vi "Read Mulit Voltage.vi"() -> ()   [LabVIEW 2019]
uses:
  BRC-DAQ.lvlib
panel:
  out "get parameters":T1={"Sample Rate"=51200.0, "Coupling Model"=1, "IEPE Current(mA)"=4.0} {"IEPE Current(mA)" format="%#_13g"; "Coupling Model" items=["DC", "AC"]; "Sample Rate" format="%#_13g"}
  out "Numeric":i32
  in  "Stop":bool
  out "Waveform Graph":waveform(dbl)[](graph)
  in  "set parameters":T1={"Sample Rate"=51200.0, "Coupling Model"=1, "IEPE Current(mA)"=4.0} {"IEPE Current(mA)" format="%#_13g"; "Coupling Model" items=["DC", "AC"]; "Sample Rate" format="%#_13g"}
  in  "Physical ID":i32
  out "Module Information":cluster{"ID":string, "Name":string, "CH":i32}[](array[cluster])
  in  "rawValue":bool
  # "Channel Setting"
  # "Acquired Data"
  # "Acquired Parameters"
  # "Module Parameters"
  # "Module Information"
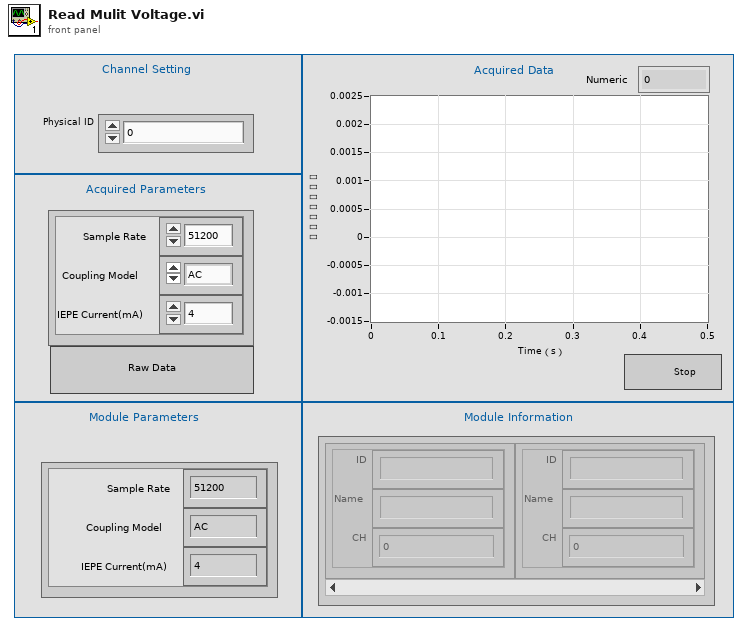
[diagram p1: front panel]
types:
  T1 = cluster{"Sample Rate":dbl, "Coupling Model":i32, "IEPE Current(mA)":dbl}
  T2 = typedef "BRC-DAQ.lvlib/brc_daq_pModuleInfo.ctl" = cluster{"deviceId":string, "productName":string, "channelCount":i32}
  T3 = cluster{"sample_rate":dbl, "coupling_mode":i32, "current":dbl}
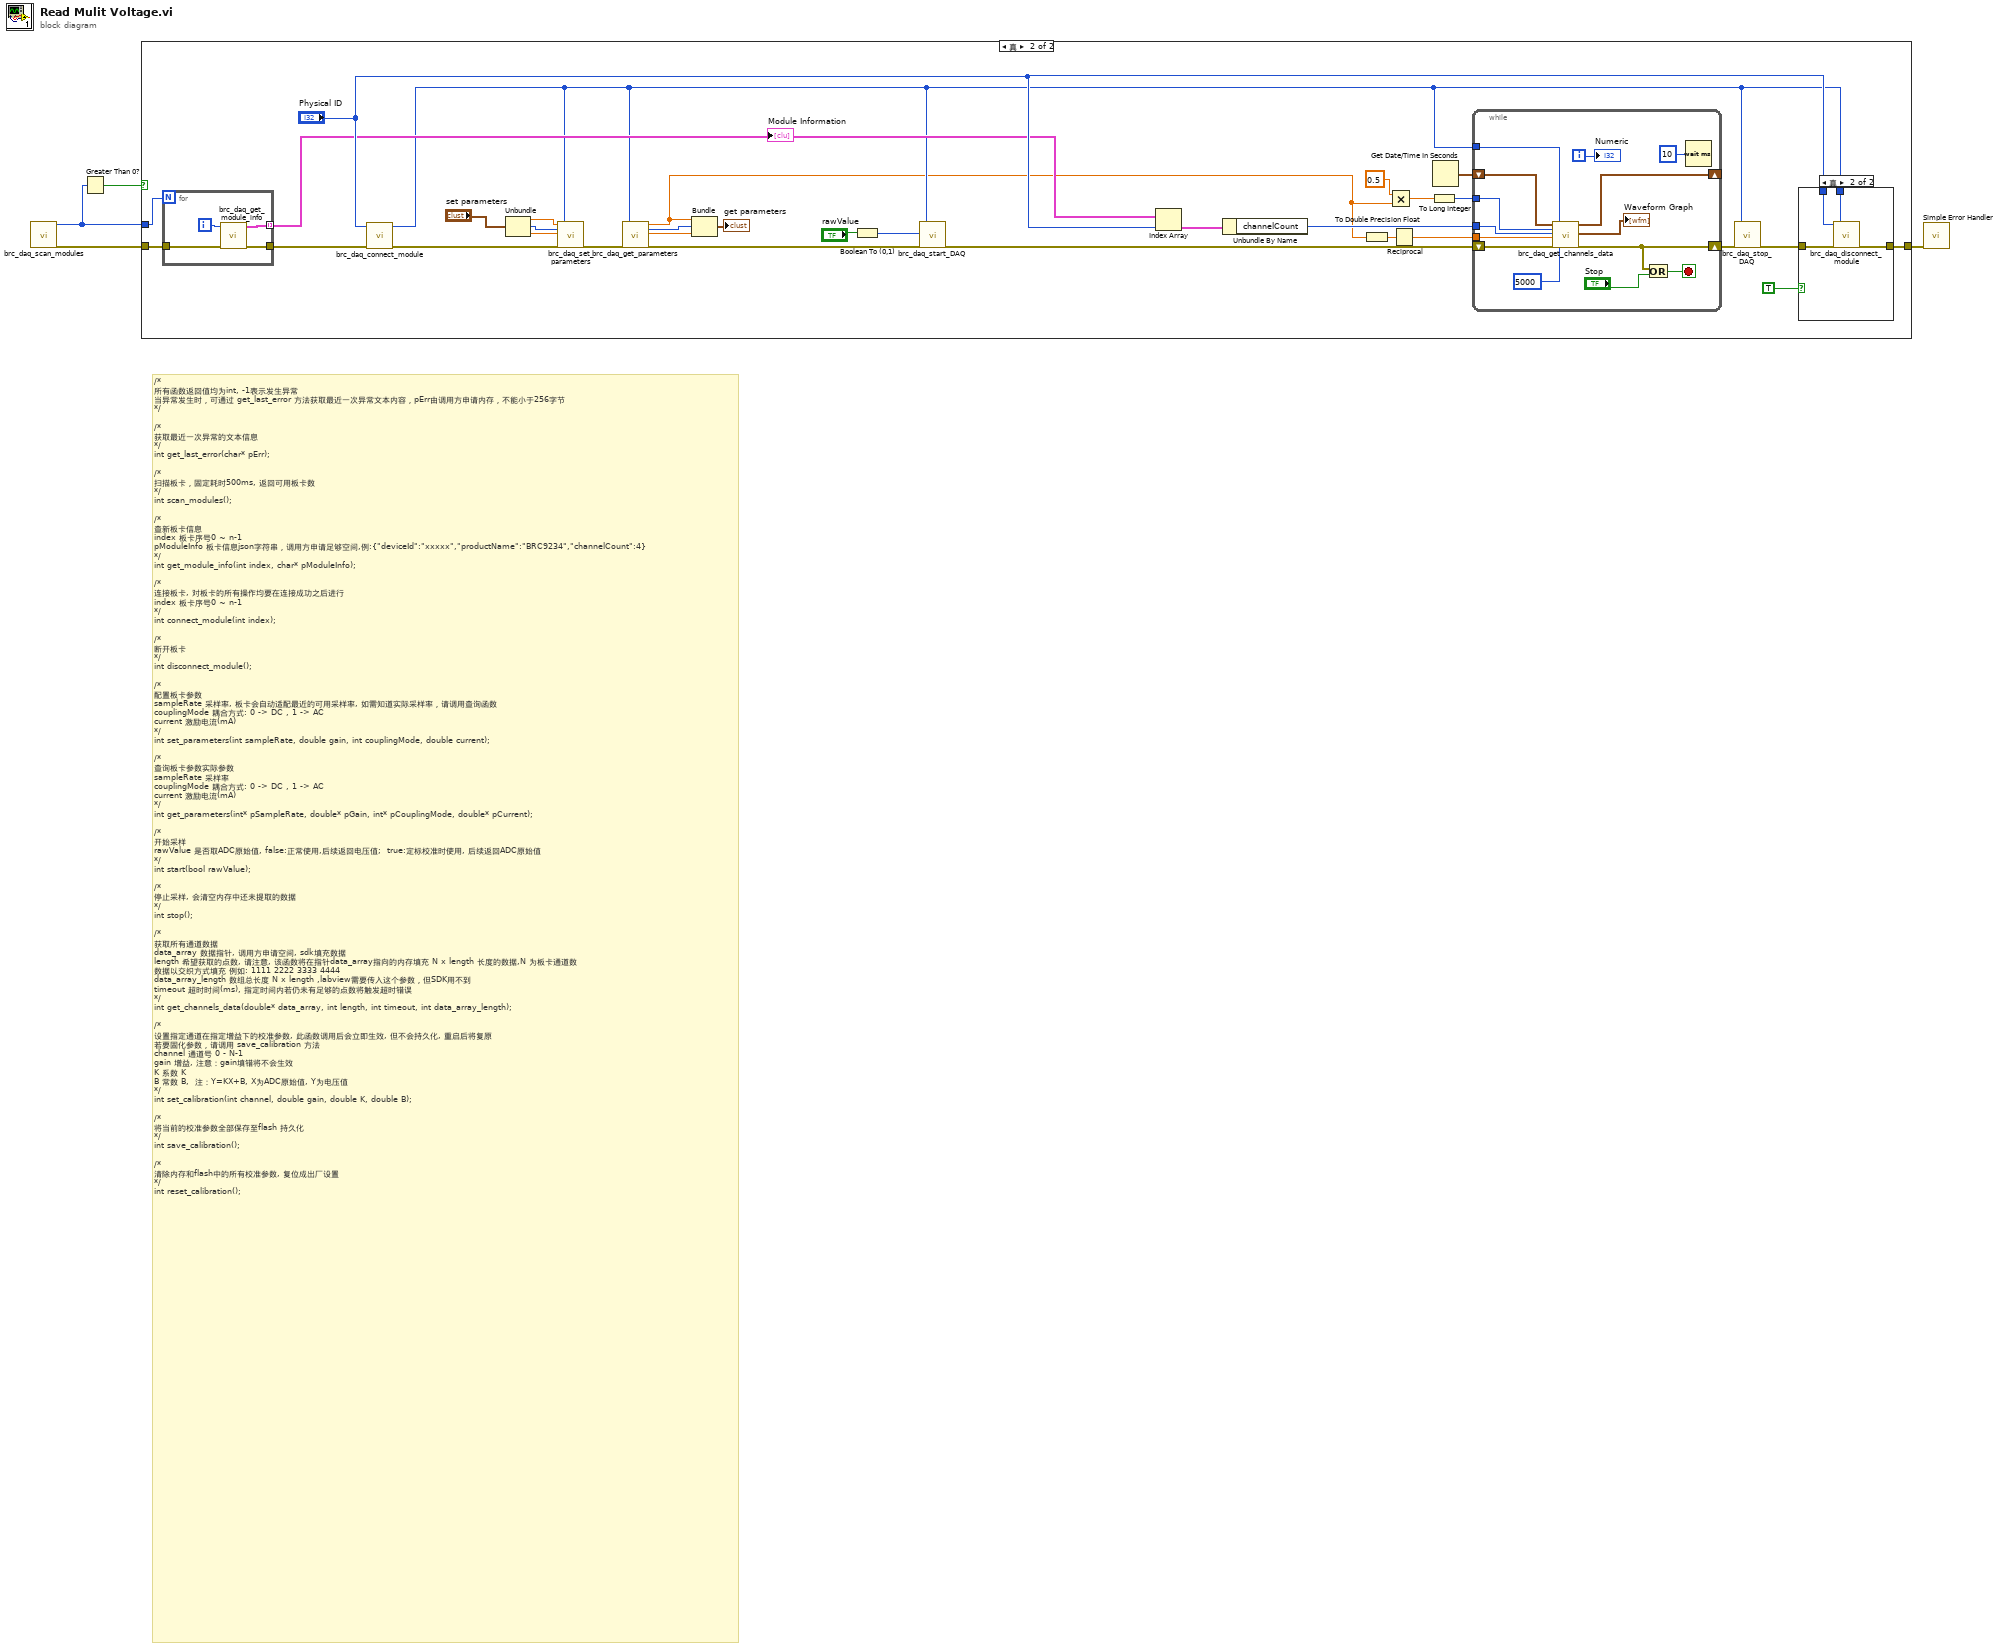
[diagram p0: block diagram]
diagram:
  # "/*\n所有函数返回值均为int, -1表示发生异常\n当异常发生时，可通过 get_last_error 方法获取最近一次异常文本内容，pErr由调用方申请内存，不能小于256字节\n*/\n\n/*\n获取最近一次异常的文本信息\n*/\nint get_last_error(char* pErr);\n\n/*\n扫描板卡，固定耗时500ms, 返回可用板卡数\n*/\nint scan_modules();\n\n/*\n查新板卡信息\nindex 板卡序号0 ~ n-1\npModuleInfo 板卡信息json字符串，调用方申请足够空间,例:{\"deviceId\":\"xxxxx\",\"productName\":\"BRC9234\",\"channelCount\":4}\n*/\nint get_module_info(int index, char* pModuleInfo);\n\n/*\n连接板卡, 对板卡的所有操作均要在连接成功之后进行\nindex 板卡序号0 ~ n-1\n*/\nint connect_module(int index);\n\n/*\n断开板卡\n*/\nint disconnect_module();\n\n/*\n配置板卡参数\nsampleRate 采样率, 板卡会自动适配最近的可用采样率, 如需知道实际采样率，请调用查询函数\ncouplingMode 耦合方式: 0 -> DC , 1 -> AC\ncurrent 激励电流(mA)\n*/\nint set_parameters(int sampleRate, double gain, int couplingMode, double current);\n\n/*\n查询板卡参数实际参数\nsampleRate 采样率\ncouplingMode 耦合方式: 0 -> DC , 1 -> AC\ncurrent 激励电流(mA)\n*/\nint get_parameters(int* pSampleRate, double* pGain, int* pCouplingMode, double* pCurrent);\n\n/*\n开始采样\nrawValue 是否取ADC原始值, false:正常使用,后续返回电压值;  true:定标校准时使用, 后续返回ADC原始值\n*/\nint start(bool rawValue);\n\n/*\n停止采样, 会清空内存中还未提取的数据\n*/\nint stop();\n\n/*\n获取所有通道数据\ndata_array 数据指针, 调用方申请空间, sdk填充数据\nlength 希望获取的点数, 请注意, 该函数将在指针data_array指向的内存填充 N x length 长度的数据,N 为板卡通道数\n数据以交织方式填充 例如: 1111 2222 3333 4444\ndata_array_length 数组总长度 N x length ,labview需要传入这个参数，但SDK用不到\ntimeout 超时时间(ms), 指定时间内若仍未有足够的点数将触发超时错误\n*/\nint get_channels_data(double* data_array, int length, int timeout, int data_array_length);\n\n/*\n设置指定通道在指定增益下的校准参数, 此函数调用后会立即生效, 但不会持久化, 重启后将复原\n若要固化参数，请调用 save_calibration 方法\nchannel 通道号 0 - N-1\ngain 增益, 注意：gain填错将不会生效\nK 系数 K\nB 常数 B,  注：Y=KX+B, X为ADC原始值, Y为电压值\n*/\nint set_calibration(int channel, double gain, double K, double B);\n\n/*\n将当前的校准参数全部保存至flash 持久化\n*/\nint save_calibration();\n\n/*\n清除内存和flash中的所有校准参数, 复位成出厂设置\n*/\nint reset_calibration();"
  n1 = call "brc_daq_scan_modules.vi"() -> ("module_number"=w2:i32, "error out"=w3:errorcluster)  [unwired: 18 in]
  n2 = Greater Than 0?(x=w2) -> (x > 0?=w1:bool)
  n3 = case shown="真" w1 {
    tunnel: w2 -> [_ w35]
    tunnel: [w5 w9] -> w4
    tunnel: w3 -> [w5 w8]
    frame False {
    }
    frame True {
      n4 = for {
        N: w35 -> [_]
        tunnel: [w60] -> w33 mode=indexing
        tunnel: w8 -> [w58]
        tunnel: [w57] -> w7
        i -> [w59]
        n5 = call "brc_daq_get_module_info.vi"("error in (no error)"=w58, "index"=w59) -> ("error out"=w57:errorcluster, "pModuleInfo_cluster"=w60:T2)  [unwired: 7 in]
      }
      "Module Information" <- w33
      n6 = call "brc_daq_connect_module.vi"("error in (no error)"=w7, "index"="Physical ID") -> ("error out"=w19:errorcluster, "return_value"=w20:i32)  [unwired: 8 in]
      n7 = Unbundle("set parameters") -> ("Sample Rate"=w16:dbl, "Coupling Model"=w15:i32, "IEPE Current(mA)"=w14:dbl)
      n8 = call "brc_daq_set_parameters.vi"("sample_rate"=w16, "coupling_mode"=w15, "current_mA"=w14, "error in (no error)"=w19, "mHandle"=w20) -> ("error out"=w28:errorcluster)  [unwired: 14 in]
      n9 = call "brc_daq_get_parameters.vi"("error in (no error)"=w28, "mHandle"=w20) -> ("sample_rate"=w13:dbl, "coupling_mode"=w12:i32, "current"=w11:dbl, "error out"=w27:errorcluster)  [unwired: 14 in]
      n10 = Bundle("sample_rate"=w13, "coupling_mode"=w12, "current"=w11) -> (→"get parameters":T3)  [unwired: 1 in]
      n11 = Boolean To (0,1)(Boolean="rawValue") -> (0, 1=w21:i16)
      n12 = call "brc_daq_start_DAQ.vi"("rawValue"=w21, "error in (no error)"=w27, "mHandle"=w20) -> ("error out"=w26:errorcluster)  [unwired: 16 in]
      n13 = Index Array(array=w33, index="Physical ID") -> (element=w36:T2)
      n14 = Unbundle By Name(w36) -> ("channelCount"=w37:i32)
      n15 = To Double Precision Float(number=w13) -> (double precision float=w30:dbl)
      n16 = Multiply(x=0.5, y=w13) -> (x*y=w32:dbl)
      n17 = Reciprocal(x=w30) -> (1/x=w29:dbl)
      n18 = To Long Integer(number=w32) -> (32bit integer=w31:i32)
      n19 = Get Date/Time In Seconds() -> (seconds since 1Jan1904=w23:timestamp)
      n20 = while {
        shift-right: [w45] -> w25
        shift-left: w26 -> [w56]
        tunnel: w31 -> [w54]
        tunnel: w37 -> [w53]
        tunnel: w29 -> [w51]
        shift-right: [w48] -> _
        shift-left: w23 -> [w49]
        tunnel: w20 -> [w47]
        i -> [w50]
        stop <- w55 stop-if-true
        n21 = call "brc_daq_get_channels_data.vi"("t0_in"=w49, "samples_per_ch"=w54, "ch_number"=w53, "dt"=w51, "error in (no error)"=w56, "mHandle"=w47, "time_out_ms"=5000) -> ("t0_out"=w48:timestamp, "data_out"=→"Waveform Graph":waveform(dbl)[], "error out"=w45:errorcluster)  [unwired: 10 in]
        n22 = Or(x=w45, y="Stop") -> (x .or. y?=w55:bool)
        n23 = Wait (ms)(milliseconds to wait=u32 10) -> ()  [unwired: 1 out]
        "Numeric" <- w50
      }
      n24 = call "brc_daq_stop_DAQ.vi"("error in (no error)"=w25, "mHandle"=w20) -> ("error out"=w24:errorcluster)  [unwired: 17 in]
      n25 = case shown="真" TRUE {
        tunnel: "Physical ID" -> [_ w42]
        tunnel: w24 -> [w38 w41]
        tunnel: w20 -> [_ w40]
        tunnel: [w38 w39] -> w9
        frame False {
        }
        frame True {
          n26 = call "brc_daq_disconnect_module.vi"("index"=w42, "error in (no error)"=w41, "mHandle"=w40) -> ("error out"=w39:errorcluster)  [unwired: 16 in]
        }
      }
    }
  }
  n27 = call <vilib>:"Simple Error Handler.vi"("error in (no error)"=w4) -> ()  [unwired: 4 in, 5 out]
